vi "BK Precision 911X Series Output DC Volts.vi"() -> ()   [LabVIEW 2019]
doc: "This example shows how to configure the instrument's output voltage level and over voltage protection. The actual voltage level and actual current level are returned."
uses:
  <instrlib>/BK Precision 911X Series/BK Precision 911X Series.lvlib
panel:
  in  "Current Limit (0.0 A)":dbl format="%.3g"
  in  "Enable OVP (T: Enable)":bool=TRUE
  in  "Stop Output":bool
  in  "Voltage Limit (0V)":dbl format="%.2f"
  out "Actual Current Limit (A)":dbl format="%.3f"
  out "Actual Voltage Level (V)":dbl format="%.3f"
  in  "Voltage Level (0.0 V)":dbl format="%.3f"
  in  "VISA resource name":refnum<visa-resource-name>
  # "(c) 2013 B&K Precision Corporation.  ALL RIGHTS RESERVED."
  # "Over Voltage Protection"
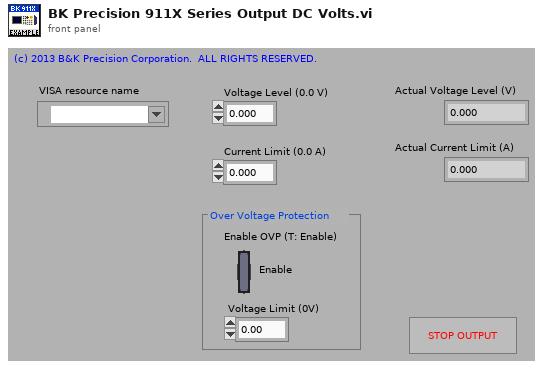
[diagram p1: front panel]
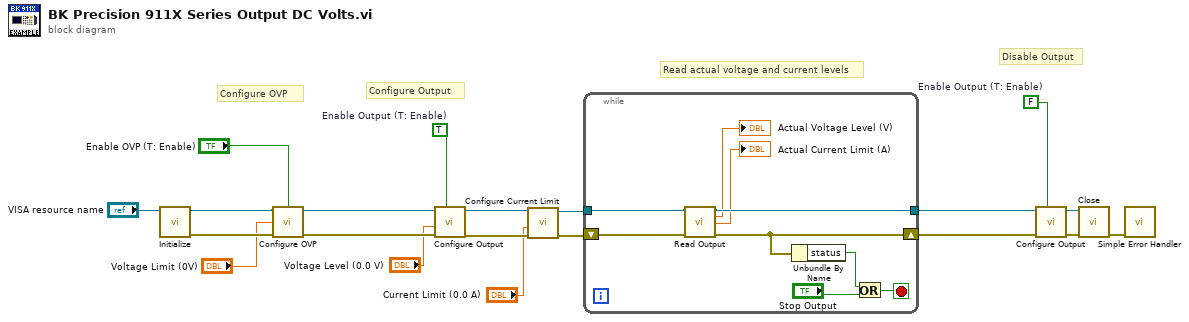
[diagram p0: block diagram]
diagram:
  w7 = FALSE  # Enable Output (T: Enable)
  w13 = TRUE  # Enable Output (T: Enable)
  # "Disable Output"
  # "Read actual voltage and current levels"
  # "Configure Output"
  # "Configure OVP"
  n1 = call <instrlib>:"Initialize.vi"("VISA resource name"="VISA resource name") -> ("error out"=w18:errorcluster, "VISA resource name out"=w17:refnum<visa-resource-name>)  [unwired: 9 in]
  n2 = call <instrlib>:"Configure OVP.vi"("VISA resource name"=w17, "Enable OVP (T: Enable)"="Enable OVP (T: Enable)", "Voltage Limit (80.000 V)"="Voltage Limit (0V)", "error in (no error)"=w18) -> ("VISA resource name out"=w15:refnum<visa-resource-name>, "error out"=w14:errorcluster)  [unwired: 10 in]
  n3 = call <instrlib>:"Configure Output.vi"("Enable Output (T: Enable)"=w13, "error in (no error)"=w14, "Voltage Level (0.0 V)"="Voltage Level (0.0 V)", "VISA resource name"=w15) -> ("error out"=w4:errorcluster, "VISA resource name out"=w5:refnum<visa-resource-name>)  [unwired: 6 in]
  n4 = call <instrlib>:"Configure Current Limit.vi"("error in (no error)"=w4, "Current Limit (0.0 A)"="Current Limit (0.0 A)", "VISA resource name"=w5) -> ("error out"=w3:errorcluster, "VISA resource name out"=w2:refnum<visa-resource-name>)  [unwired: 7 in]
  n5 = while {
    tunnel: w2 -> [w26]
    tunnel: [w23] -> w11
    shift-right: [w24] -> w10
    shift-left: w3 -> [w25]
    stop <- w29 stop-if-true
    n6 = call <instrlib>:"Read Output.vi"("VISA resource name"=w26, "error in (no error)"=w25) -> ("VISA resource name out"=w23:refnum<visa-resource-name>, "Actual Voltage Level (V)"=→"Actual Voltage Level (V)":dbl, "Actual Current Level (A)"=→"Actual Current Limit (A)":dbl, "error out"=w24:errorcluster)  [unwired: 8 in, 2 out]
    n7 = Unbundle By Name(w24) -> ("status"=w27:bool)
    n8 = Or(x=w27, y="Stop Output") -> (x .or. y?=w29:bool)
  }
  n9 = call <instrlib>:"Configure Output.vi"("Enable Output (T: Enable)"=w7, "error in (no error)"=w10, "VISA resource name"=w11) -> ("error out"=w8:errorcluster, "VISA resource name out"=w9:refnum<visa-resource-name>)  [unwired: 7 in]
  n10 = call <instrlib>:"Close.vi"("error in (no error)"=w8, "VISA resource name"=w9) -> ("error out"=w19:errorcluster)  [unwired: 9 in]
  n11 = call <vilib>:"Simple Error Handler.vi"("error in (no error)"=w19) -> ()  [unwired: 4 in, 5 out]
